vi "close_DLP_.vi"(8 "error in (no error)":errorcluster, 10 "SequenceId":u32, 11 "DeviceId":u32) -> (0 "error out":errorcluster)   [LabVIEW 2020]
uses:
  <vilib>/Utility/error.llb/Error Cluster From Error Code.vi
  <userlib>/alp4395/alp4395.dll
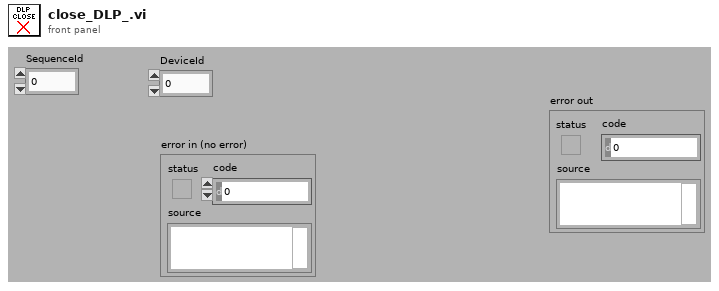
[diagram p1: front panel]
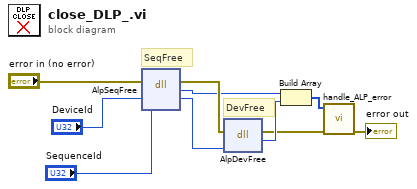
[diagram p0: block diagram]
diagram:
  # "SeqFree"
  # "DevFree"
  n1 = dll-call lib="C:/Program Files (x86)/National Instruments/LabVIEW 2020/user.lib/alp4395/alp4395.dll" fn="AlpSeqFree"(error in="error in (no error)", "DeviceId"="DeviceId", "SequenceId"="SequenceId") -> (error out=w10:errorcluster, "return type"=w5:i32, "DeviceId"=w9:u32)  [unwired: 3 in, 1 out]
  n2 = dll-call lib="C:/Program Files (x86)/National Instruments/LabVIEW 2020/user.lib/alp4395/alp4395.dll" fn="AlpDevFree"(error in=w10, "DeviceId"=w9) -> (error out=w3:errorcluster, "return type"=w4:i32)  [unwired: 3 in, 1 out]
  n3 = Build Array(w5, w4) -> (w6:i32[])
  n4 = call "handle_ALP_error.vi"("error in"=w3, "Return Codes"=w6) -> ("error out"=→"error out":errorcluster)  [unwired: 9 in]
